vi "Process Point Defense.vi"(11 "Chmmr in":refnum<class "Chmmr.lvclass">) -> (3 "Chmmr out":refnum<class "Chmmr.lvclass">)   [LabVIEW 2021, in "Chmmr.lvclass"]
uses:
  Chmmr.lvclass
  Chmmr.lvclass/Chmmr.ctl
  Element/Element.lvclass
  Globals.vi
  Vector 2D/Vector 2D.lvclass
panel:
  in  "Satellites.Max Hit Distance":i32=256
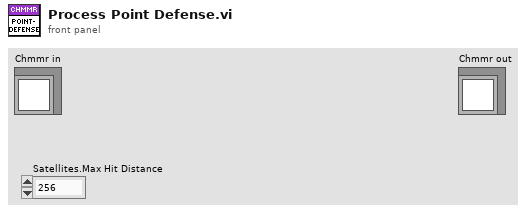
[diagram p1: front panel]
types:
  T1 = typedef "Element.lvclass/Player Type.ctl" = enum16{"Neutral", "Player 1", "Player 2"}
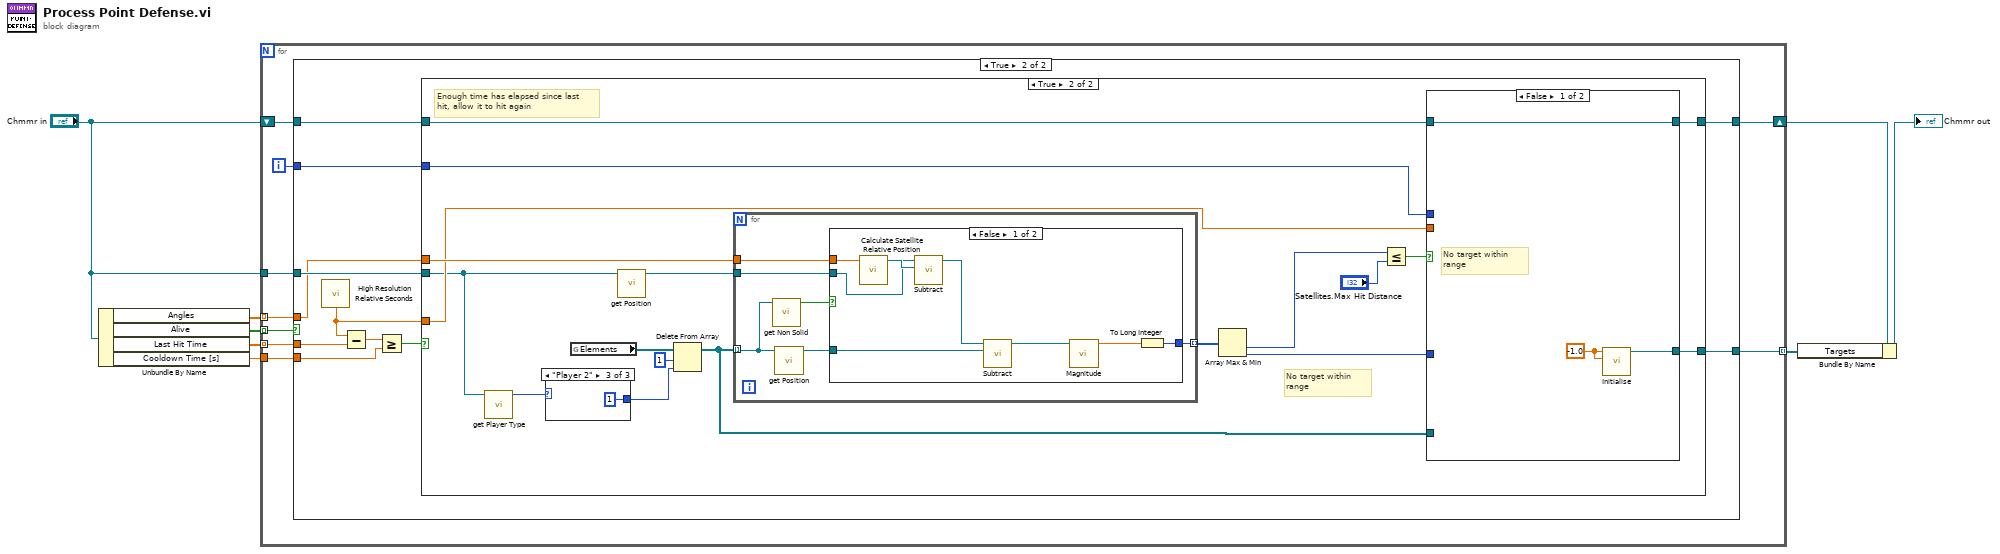
[diagram p0: block diagram]
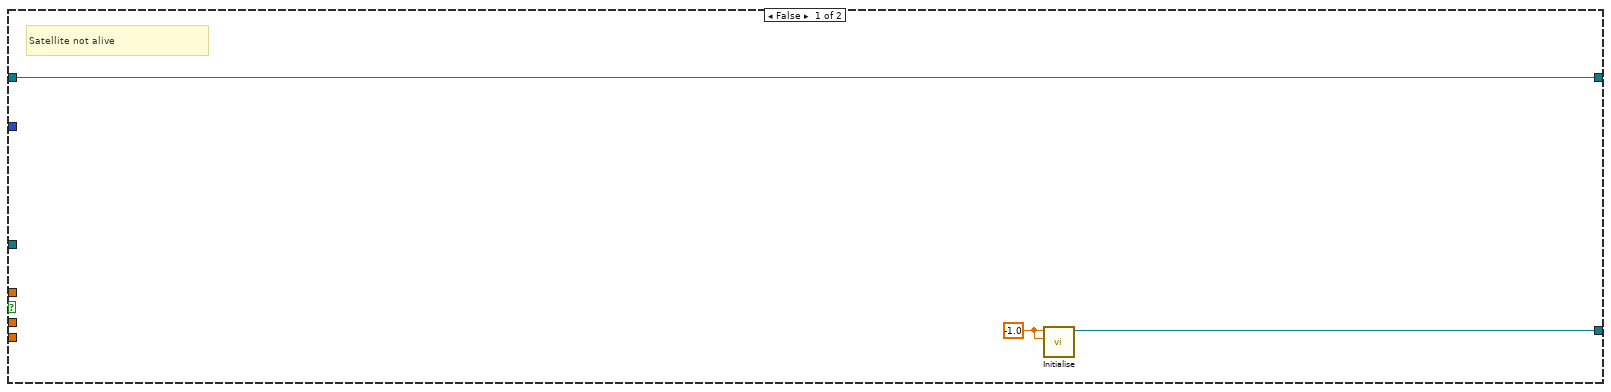
[diagram p2: hidden frame]
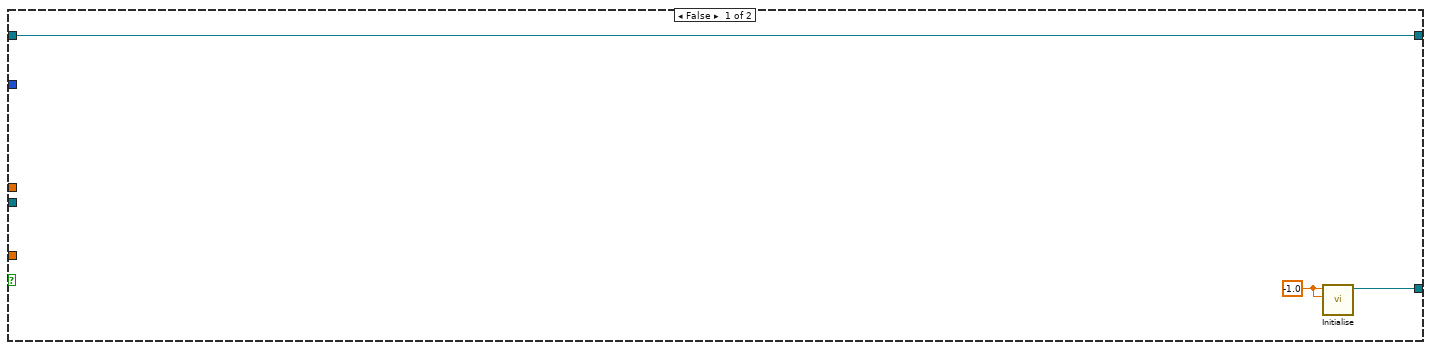
[diagram p3: hidden frame]
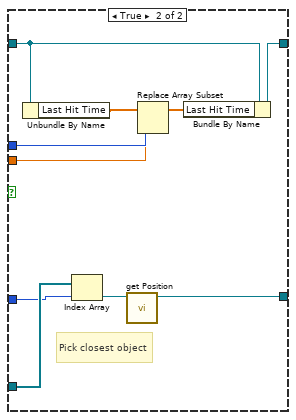
[diagram p4: hidden frame]
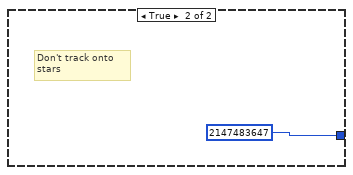
[diagram p5: hidden frame]
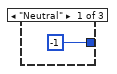
[diagram p6: hidden frame]
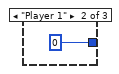
[diagram p7: hidden frame]
diagram:
  n1 = Unbundle By Name("Chmmr in") -> ("Angles"=w5:sgl[], "Alive"=w7:bool[], "Last Hit Time"=w4:dbl[], "Cooldown Time [s]"=w3:dbl)
  n2 = for {
    tunnel: "Chmmr in" -> [w17]
    tunnel: w7 -> [w16] mode=indexing
    tunnel: [w15] -> w6 mode=indexing
    tunnel: w5 -> [w14] mode=indexing
    tunnel: w4 -> [w13] mode=indexing
    tunnel: w3 -> [w12]
    shift-right: [w10] -> w2
    shift-left: "Chmmr in" -> [w11]
    i -> [w9]
    n3 = case shown="True" w16 {
      tunnel: w17 -> [_ w31]
      tunnel: [w18 w30] -> w15
      tunnel: w14 -> [_ w29]
      tunnel: w13 -> [_ w28]
      tunnel: w12 -> [_ w26]
      tunnel: w11 -> [w20 w25]
      tunnel: [w20 w24] -> w10
      tunnel: w9 -> [_ w23]
      frame False {
        w19 = sgl -1.0 ("x")
        # "Satellite not alive"
        n4 = call "Initialise.vi"("y"=w19, "x"=w19) -> ("Vector 2D out"=w18:refnum<class "Vector 2D.lvclass">)  [unwired: 9 in]
      }
      frame True {
        n5 = call <vilib>:"High Resolution Relative Seconds.vi"() -> ("relative seconds"=w22:dbl)
        n6 = Subtract(x=w22, y=w28) -> (x-y=w27:dbl)
        n7 = Greater Or Equal?(x=w27, y=w26) -> (x >= y?=w21:bool)
        n8 = case shown="True" w21 {
          tunnel: w31 -> [_ w36]
          tunnel: [w32 w47] -> w30
          tunnel: w29 -> [_ w41]
          tunnel: w25 -> [w34 w40]
          tunnel: [w34 w39] -> w24
          tunnel: w23 -> [_ w38]
          tunnel: w22 -> [_ w37]
          frame False {
            w33 = sgl -1.0 ("x")
            n9 = call "Initialise.vi"("y"=w33, "x"=w33) -> ("Vector 2D out"=w32:refnum<class "Vector 2D.lvclass">)  [unwired: 9 in]
          }
          frame True {
            # "Enough time has elapsed since last hit, allow it to hit again"
            # "No target within range"
            n10 = call "get Player Type.vi"("Element in"=w36) -> ("Player Type"=w51:T1)  [unwired: 10 in]
            n11 = case shown="\"Player 2\"" w51 {
              tunnel: [-1 0 1] -> w49
              frame "Neutral" {
              }
              frame "Player 1" {
              }
              frame "Player 2" {
              }
            }
            n12 = global read "Globals.vi" "Elements"() -> (w52:refnum<class "Element.lvclass">[])
            n13 = call "get Position.vi"("Element in"=w36) -> ("Position"=w35:refnum<class "Vector 2D.lvclass">)  [unwired: 10 in]
            n14 = Delete From Array(array=w52, length=1, index=w49) -> (array with subset deleted=w43:refnum<class "Element.lvclass">[])  [unwired: 1 out]
            n15 = for {
              tunnel: w43 -> [w67] mode=indexing
              tunnel: w35 -> [w71]
              tunnel: [w70] -> w48 mode=indexing
              tunnel: w41 -> [w68]
              n16 = call "get Non Solid.vi"("Element in"=w67) -> ("Non Solid"=w69:bool)  [unwired: 10 in]
              n17 = call "get Position.vi"("Element in"=w67) -> ("Position"=w66:refnum<class "Vector 2D.lvclass">)  [unwired: 10 in]
              n18 = case shown="False" w69 {
                tunnel: w71 -> [w76 _]
                tunnel: w66 -> [w74 _]
                tunnel: [w79 2147483647] -> w70
                tunnel: w68 -> [w78 _]
                frame False {
                  n19 = call "Calculate Satellite Relative Position.vi"("Angle [deg]"=w78) -> ("Position"=w77:refnum<class "Vector 2D.lvclass">)  [unwired: 10 in]
                  n20 = call "Subtract.vi"("B"=w77, "A"=w76) -> ("A-B"=w75:refnum<class "Vector 2D.lvclass">)  [unwired: 9 in]
                  n21 = call "Subtract.vi"("B"=w74, "A"=w75) -> ("A-B"=w72:refnum<class "Vector 2D.lvclass">)  [unwired: 9 in]
                  n22 = call "Magnitude.vi"("A"=w72) -> ("Magnitude"=w73:sgl)  [unwired: 10 in]
                  n23 = To Long Integer(number=w73) -> (32bit integer=w79:i32)
                }
                frame True {
                  # "Don't track onto stars"
                }
              }
            }
            n24 = Array Max & Min(array=w48) -> (min value=w45:i32, min index (indices)=w42:i32)  [unwired: 2 out]
            n25 = Less Or Equal?(x=w45, y="Satellites.Max Hit Distance") -> (x <= y?=w44:bool)
            n26 = case shown="False" w44 {
              tunnel: [w54 w56] -> w47
              tunnel: w43 -> [_ w65]
              tunnel: w42 -> [_ w64]
              tunnel: w40 -> [w55 w62]
              tunnel: [w55 w63] -> w39
              tunnel: w38 -> [_ w59]
              tunnel: w37 -> [_ w58]
              frame False {
                w53 = sgl -1.0 ("x")
                # "No target within range"
                n27 = call "Initialise.vi"("y"=w53, "x"=w53) -> ("Vector 2D out"=w54:refnum<class "Vector 2D.lvclass">)  [unwired: 9 in]
              }
              frame True {
                # "Pick closest object"
                n28 = Unbundle By Name(w62) -> ("Last Hit Time"=w61:dbl[])
                n29 = Index Array(array=w65, index=w64) -> (element=w57:refnum<class "Element.lvclass">)
                n30 = call "get Position.vi"("Element in"=w57) -> ("Position"=w56:refnum<class "Vector 2D.lvclass">)  [unwired: 10 in]
                n31 = Replace Array Subset(array=w61, new element=w58, index=w59) -> (w60:dbl[])
                n32 = Bundle By Name(cluster=w62, "Last Hit Time"=w60) -> (w63:refnum<class "Chmmr.lvclass">)
              }
            }
          }
        }
      }
    }
  }
  n33 = Bundle By Name(cluster=w2, "Targets"=w6) -> (→"Chmmr out":refnum<class "Chmmr.lvclass">)
